vi "Dir Watch.vi"() -> ()   [LabVIEW 2019]
panel:
  in  "Files":i32(listbox) caption="Files (Only files are shown, not folders)"
  in  "stop":bool
  in  "Watch Directory":path
  # "Set \"Watch Directory\" then run this vi. The \"Files\" listbox\nwill update with the files in that directory. Add or delete\nfiles in Watch Directory using Windows Explorer and the\nlistbox will automatically update. A better demo would\nbe to use a tree control but this demonstrates the basics."
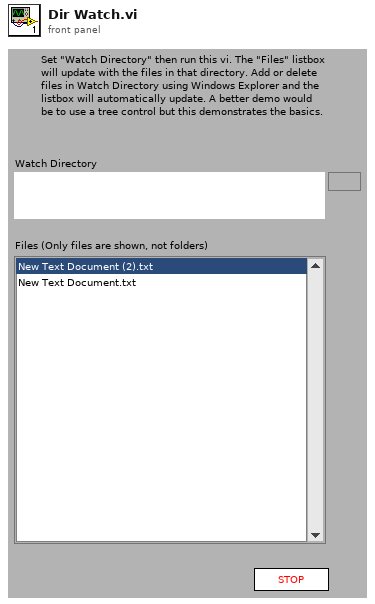
[diagram p1: front panel]
types:
  T1 = cluster{"Dir Event":refnum<user-event>, "Watch Directory":path}
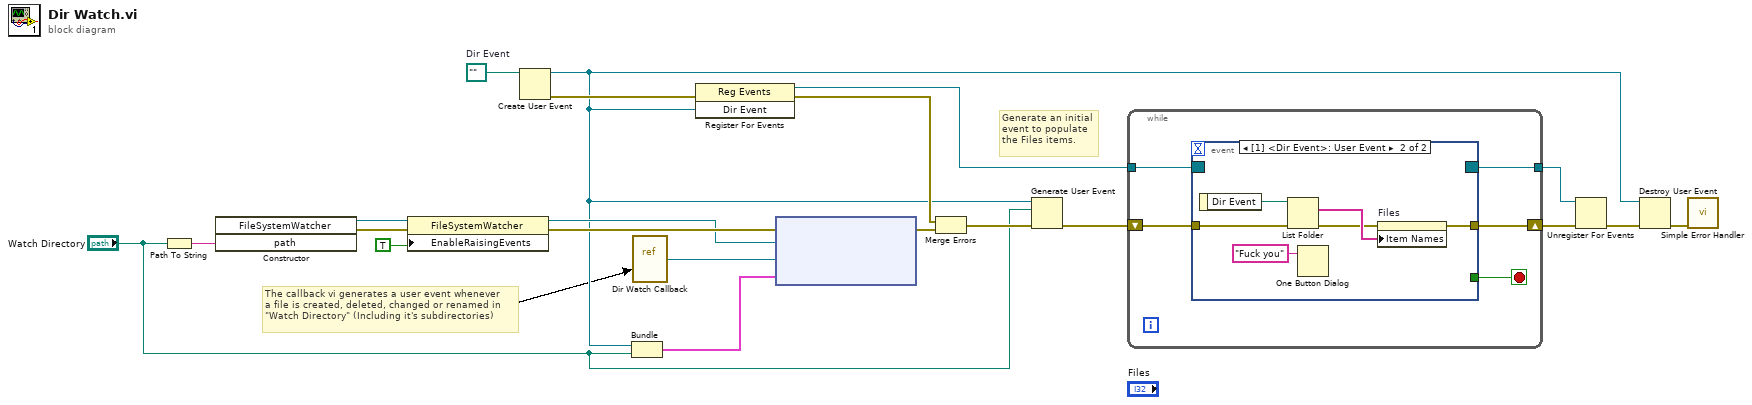
[diagram p0: block diagram]
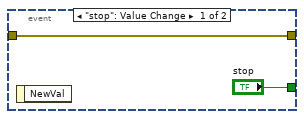
[diagram p2: hidden frame]
diagram:
  w5 = path ""  # Dir Event
  # "Generate an initial\nevent to populate\nthe Files items."
  # "The callback vi generates a user event whenever\na file is created, deleted, changed or renamed in\n\"Watch Directory\" (Including it's subdirectories)"
  n1 = Path To String(path="Watch Directory") -> (string=w17:string)
  n2 = constructor class="FileSystemWatcher"("path"=w17) -> (reference out=w20:refnum<k24>, error out=w18:errorcluster)  [unwired: 3 in, 2 out]
  n3 = property class="FileSystemWatcher"(reference=w20, error in=w18, "EnableRaisingEvents"=TRUE) -> (reference out=w8:refnum<k24>, error out=w21:errorcluster)
  n4 = Create User Event(user event datatype=w5) -> (user event=w2:refnum<user-event>, error out=w16:errorcluster)  [unwired: 1 in]
  n5 = Bundle("Dir Event"=w2, "Watch Directory"="Watch Directory") -> (w7:T1)  [unwired: 1 in]
  n6 = vi-ref "Dir Watch Callback.vi"() -> ("vi reference"=w6:refnum<vi>)
  n7 = register-events(error in=w16, w2) -> (reference out=w9:refnum<event-registration>, error out=w14:errorcluster)  [unwired: 1 in]
  n8 = node(w21, w8, w6, w7) -> (w15:errorcluster)  [unwired: 1 in, 1 out]
  n9 = Merge Errors(w14, w15) -> (w4:errorcluster)
  n10 = Generate User Event(user event=w2, event data cluster="Watch Directory", error in=w4) -> (error out=w3:errorcluster)  [unwired: 1 in, 1 out]
  n11 = while {
    tunnel: w9 -> [w25]
    shift-right: [w23] -> w12
    shift-left: w3 -> [w24]
    tunnel: [w22] -> w13
    stop <- w26 stop-if-true
    n12 = event shown="[1] <Dir Event>: User Event" {
      selector: w25 -> [_ _]
      dyn-events: [_ _] -> w22
      timeout: _ -> [_ _]
      tunnel: ["stop" _] -> w26
      tunnel: w24 -> [w27 w34]
      tunnel: [w27 w30] -> w23
      event "stop": Value Change {
        n13 = event-data() -> ()  [unwired: 1 in, 1 out]
      }
      event User Event {
        n14 = event-data() -> ("Dir Event"=w33:path)  [unwired: 1 in]
        n15 = List Folder(path=w33, error in=w34) -> (filenames=w32:string[], error out=w31:errorcluster)  [unwired: 2 in, 2 out]
        n16 = One Button Dialog(message="Fuck you") -> ()  [unwired: 1 in, 1 out]
        n17 = property on="Files" class="LstBox (strict)"(error in=w31, "Item Names"=w32) -> (error out=w30:errorcluster)  [unwired: 1 in, 1 out]
      }
    }
  }
  n18 = Unregister For Events(event registration refnum=w13, error in=w12) -> (error out=w11:errorcluster)
  n19 = Destroy User Event(user event=w2, error in=w11) -> (error out=w10:errorcluster)
  n20 = call <vilib>:"Simple Error Handler.vi"("error in (no error)"=w10) -> ()  [unwired: 4 in, 5 out]
